vi "methane_reactor_run.vi"(10 "spec_file":path) -> (2 "methane_path":path)   [LabVIEW 2019]
uses:
  <vilib>/Utility/sysdir.llb/System Directory Type.ctl
  lib/libSimulationControl/libSimulationControl.lvlib
panel:
  out "standard output":string
  out "standard error":string
  # "*******************************************************************\nBiogas Plant Control\n\nAuthor: Paul Zügel\nGCSC-Frankfurt am Main 2020\n\n*******************************************************************"
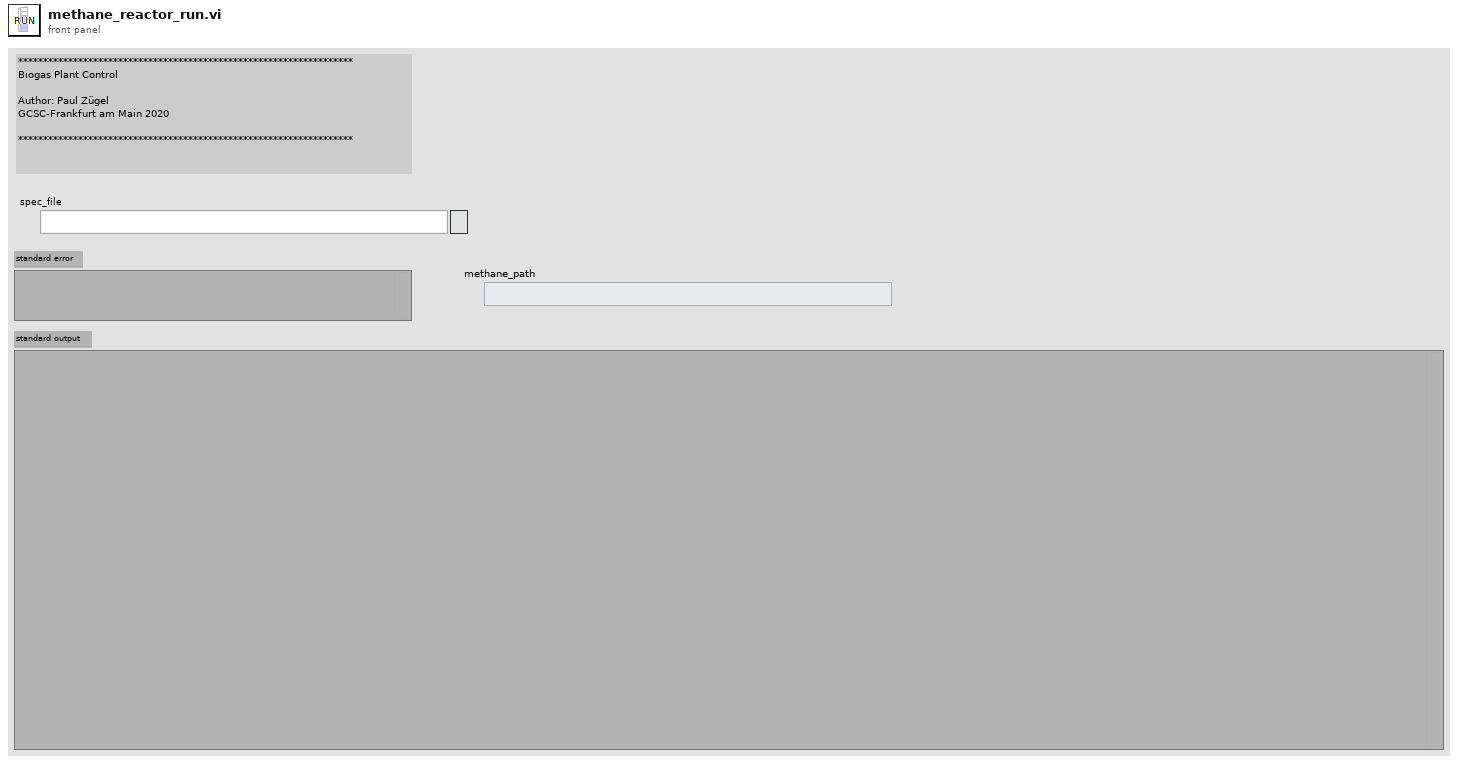
[diagram p1: front panel]
types:
  T1 = typedef "System Directory Type.ctl" = i32
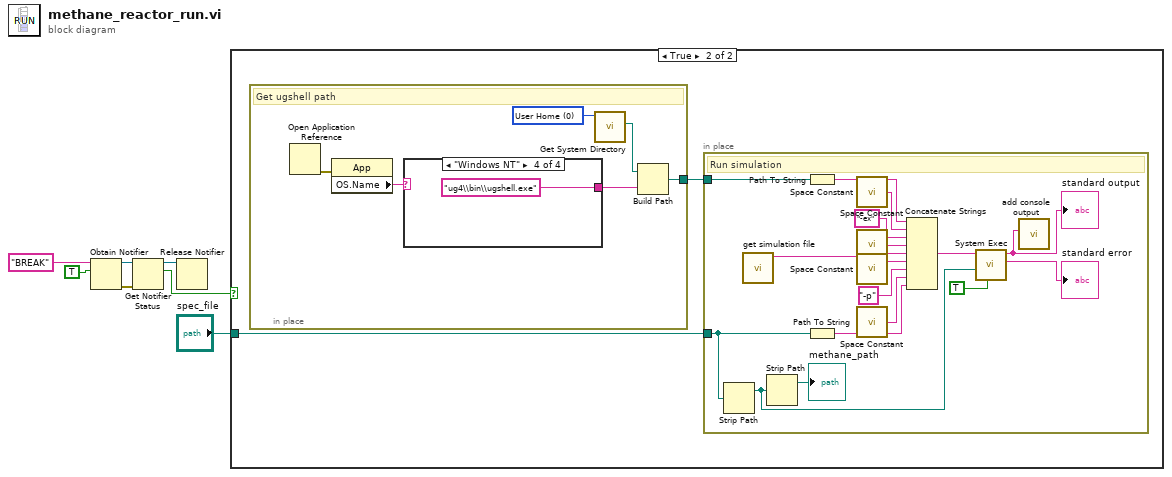
[diagram p0: block diagram]
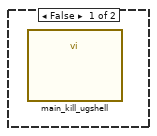
[diagram p2: hidden frame]
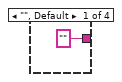
[diagram p3: hidden frame]
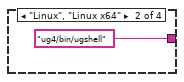
[diagram p4: hidden frame]
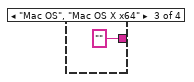
[diagram p5: hidden frame]
diagram:
  n1 = Obtain Notifier(name (unnamed)="BREAK", notification data type=TRUE) -> (notifier out=w5:refnum<notifier>, error out=w4:errorcluster)  [unwired: 2 in, 1 out]
  n2 = Get Notifier Status(notifier=w5, error in (no error)=w4) -> (notifier out=w1:refnum<notifier>, current notification=w3:bool)  [unwired: 3 out]
  n3 = Release Notifier(notifier=w1) -> ()  [unwired: 2 in, 3 out]
  n4 = case shown="True" w3 {
    tunnel: "spec_file" -> [_ w8]
    frame False {
      n5 = call "main_kill_ugshell.vi"() -> ()  [unwired: 12 in]
    }
    frame True {
      # "True only on first Iteration (current_time = starttime)\nWe get all names of output Files from the outputFiles.lua and copy them from tmp to the working directory."
      n6 = in-place {
        in-place-border: [w31] -> w9
        w30 = T1 0 items=["User Home"=0, "User Desktop"=1, "User Documents"=2, "User Application Data"=3, "User Preferences"=4, "User Temporary"=5, "Public Documents"=6, "Public Application Data"=7, "Public Preferences"=8, "Public Cache"=13, "System Core Libraries"=9, "System Installed Libraries"=10, "Application Files"=11, "Boot Volume Root"=12] ("system directory type")
        # "Get ugshell path"
        n7 = Open Application Reference() -> (0:w28:errorcluster)  [unwired: 4 in, 1 out]
        n8 = property class="App"(error in=w28) -> ("OS.Name"=w29:string)  [unwired: 1 in, 2 out]
        n9 = case shown="\"Windows NT\"" w29 {
          tunnel: ["" ("return type") "ug4/bin/ugshell" ("name or relative path") "" ("return type") "ug4\\bin\\ugshell.exe" ("name or relative path")] -> w27
          frame "", Default {
          }
          frame "Linux", "Linux x64" {
          }
          frame "Mac OS", "Mac OS X x64" {
          }
          frame "Windows NT" {
          }
        }
        n10 = call <vilib>:"Get System Directory.vi"("system directory type"=w30) -> ("system directory"=w32:path)  [unwired: 10 in]
        n11 = Build Path(base path=w32, name or relative path=w27) -> (appended path=w31:path)
      }
      n12 = in-place {
        in-place-border: w9 -> [w22]
        in-place-border: w8 -> [w12]
        # "Run simulation"
        n13 = Strip Path(path=w12) -> (stripped path=w11:path)  [unwired: 1 out]
        n14 = call "get simulation file.vi"() -> ("function return"=w15:string)  [unwired: 10 in, 1 out]
        n15 = Strip Path(path=w11) -> (stripped path=→"methane_path":path)  [unwired: 1 out]
        n16 = Path To String(path=w22) -> (string=w18:string)
        n17 = Path To String(path=w12) -> (string=w13:string)
        n18 = call <vilib>:"Space Constant.vi"() -> ("String"=w19:string)
        n19 = call <vilib>:"Space Constant.vi"() -> ("String"=w20:string)
        n20 = call <vilib>:"Space Constant.vi"() -> ("String"=w21:string)
        n21 = call <vilib>:"Space Constant.vi"() -> ("String"=w24:string)
        n22 = Concatenate Strings(w18, w19, "-ex" ("command line"), w20, w15, w21, "-p" ("command line"), w24, w13) -> (w23:string)
        n23 = call <vilib>:"System Exec.vi"("run minimized? (F)"=TRUE, "working directory"=w11, "command line"=w23) -> ("standard error"=→"standard error":string, "standard output"=w26:string)  [unwired: 5 in, 2 out]
        "standard output" <- w26
        n24 = call "add console output.vi"("add_to_console"=w26) -> ()  [unwired: 11 in]
      }
    }
  }
